vi "Vision Processor.vi"(5 "error in":errorcluster, 7 "Image In":T1) -> (0 "error out":errorcluster, 3 "Image Out":T1(plugin-control))   [LabVIEW 2014]
uses:
  <vilib>/vision/Image Controls.llb/IMAQ Image.ctl
  <vilib>/vision/NI_Vision_Development_Module.lvlib
panel:
  in  "Red or Hue Range":cluster{"Lower value":i32, "Upper value":i32}={"Lower value"=0, "Upper value"=40}
  in  "Blue or Luma or Val or Inten Range":cluster{"Lower value":i32, "Upper value":i32}={"Lower value"=0, "Upper value"=47}
  in  "Green or Sat Range":cluster{"Lower value":i32, "Upper value":i32}={"Lower value"=0, "Upper value"=226}
  out "Pre-Process":T1(plugin-control)
  # "0  center of mass x\n1  center of mass y\n2  first pixel x\n3  first pixel y\n4  bounding rect left\n5  bounding rect top\n6  bounding rect right\n7  bounding rect bottom\n8 max feret diameter start x\n9  max feret diameter start y\n10 max feret diameter end x\n11 max feret diameter end y\n12 max horiz segment length left\n13 max horiz segment length right\n14 max horiz segment length row\n15 bounding rect width \n16 bounding rect height\n17 bounding rect diagional\n..\n33 area"
  # "13'3\"\n3'9\""
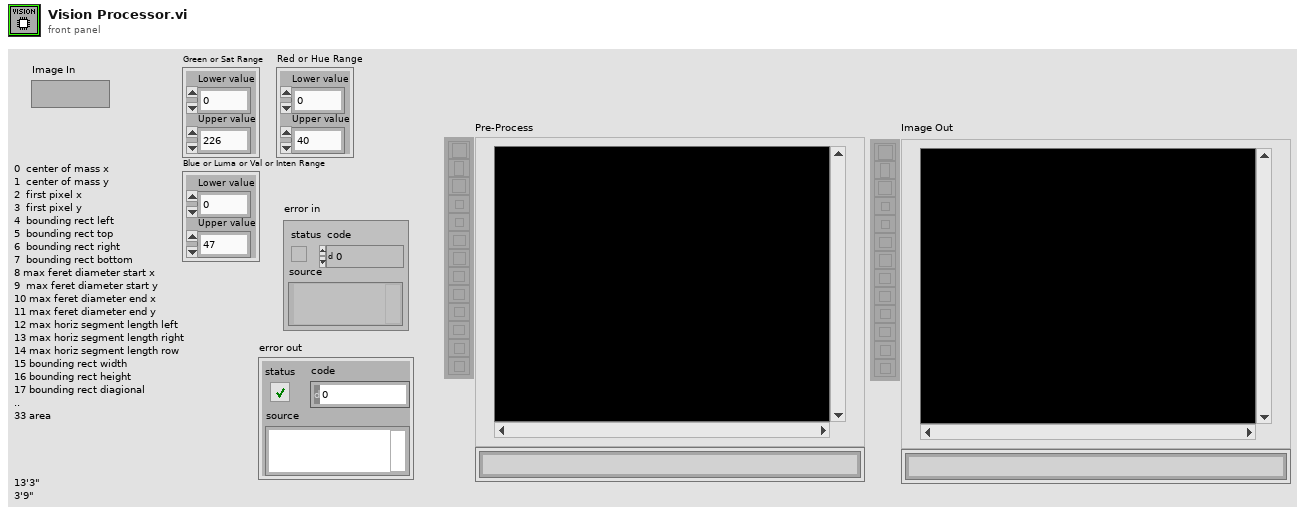
[diagram p1: front panel]
types:
  T1 = typedef "IMAQ Image.ctl" = refnum<image>
  T2 = typedef "Image Type" = u32
  T3 = enum32{"AutoM", "Close", "Dilate", "Erode", "Gradient", "Gradient out", "Gradient in", "Hit miss", "Open", "PClose", "POpen", "Thick", "Thin"}
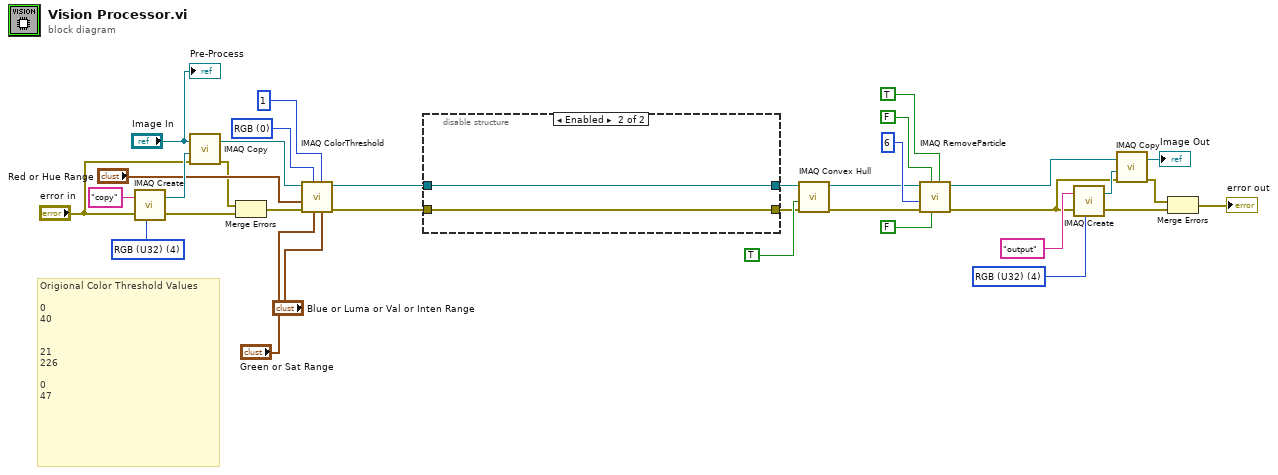
[diagram p0: block diagram]
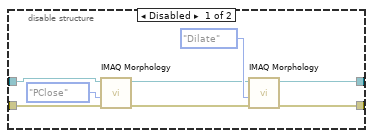
[diagram p2: hidden frame]
diagram:
  w19 = T2 4 items=["Grayscale (U8)", "Grayscale (I16)", "Grayscale (SGL)", "Complex (CSG)", "RGB (U32)", "HSL (U32)", "RGB (U64)", "Grayscale (U16)"] ("Image Type")
  w25 = T2 4 items=["Grayscale (U8)", "Grayscale (I16)", "Grayscale (SGL)", "Complex (CSG)", "RGB (U32)", "HSL (U32)", "RGB (U64)", "Grayscale (U16)"] ("Image Type")
  w32 = u16 0 items=["RGB", "HSL", "HSV", "HSI"] ("Color Mode")
  # "Origional Color Threshold Values\n\n0\n40\n\n\n21\n226\n\n0\n47"
  n1 = call "IMAQ Create"("Image Name"="copy", "Image Type"=w25, "error in (no error)"="error in") -> ("New Image"=w24:T1, "error out"=w9:errorcluster)  [unwired: 2 in]
  n2 = call "IMAQ Copy"("error in (no error)"="error in", "Image Dst"=w24, "Image Src"="Image In") -> ("error out"=w8:errorcluster, "Image Dst Out"=w1:T1)  [unwired: 3 in]
  n3 = Merge Errors(w8, w9) -> (w7:errorcluster)
  n4 = call "IMAQ ColorThreshold"("Blue or Luma or Val or Inten Range"="Blue or Luma or Val or Inten Range", "Replace Value"=1, "Green or Sat Range"="Green or Sat Range", "Color Mode"=w32, "error in (no error)"=w7, "Red or Hue Range"="Red or Hue Range", "Image Src"=w1) -> ("error out"=w22:errorcluster, "Image Dst Out"=w23:T1)  [unwired: 1 in, 2 out]
  n5 = disable-structure shown="Enabled" {
    disable-tunnel: w23 -> [w41 w44]
    disable-tunnel: w22 -> [w40 w43]
    disable-tunnel: [w36 w44] -> w15
    disable-tunnel: [w35 w43] -> w14
    frame Disabled {
      n6 = call "IMAQ Morphology"("error in (no error)"=w40, "Operation"=T3."PClose", "Image Src"=w41) -> ("error out"=w38:errorcluster, "Image Dst Out"=w37:T1)  [unwired: 7 in]
      n7 = call "IMAQ Morphology"("error in (no error)"=w38, "Operation"=T3."Dilate", "Image Src"=w37) -> ("error out"=w35:errorcluster, "Image Dst Out"=w36:T1)  [unwired: 7 in]
    }
    frame Enabled {
    }
  }
  n8 = call "IMAQ Convex Hull"("error in (no error)"=w14, "Connectivity 4/8 (8)"=TRUE, "Image Src"=w15) -> ("error out"=w21:errorcluster, "Image Dst Out"=w20:T1)  [unwired: 1 in, 6 out]
  n9 = call "IMAQ RemoveParticle"("Connectivity 4/8 (8)"=TRUE, "Low Pass/High Pass (Low)"=FALSE, "Square/Hexa (Square)"=FALSE, "error in (no error)"=w21, "Number of Erosion"=6, "Image Src"=w20) -> ("error out"=w10:errorcluster, "Image Dst Out"=w16:T1)  [unwired: 1 in, 3 out]
  n10 = call "IMAQ Create"("Image Name"="output", "Image Type"=w19, "error in (no error)"=w10) -> ("New Image"=w17:T1, "error out"=w6:errorcluster)  [unwired: 2 in]
  n11 = call "IMAQ Copy"("error in (no error)"=w10, "Image Dst"=w17, "Image Src"=w16) -> ("error out"=w5:errorcluster, "Image Dst Out"=→"Image Out":T1)  [unwired: 3 in]
  n12 = Merge Errors(w5, w6) -> (→"error out":errorcluster)
  "Pre-Process" <- "Image In"
